vi "XboxControl.vi"() -> ()   [LabVIEW 2011]
uses:
  <vilib>/Utility/inputDevices.llb/joystickAcquire.vi
panel:
  out "A Speed Value":dbl
  in  "stop":bool
  out "direction info":T1
  out "button info":T2
  out "axis info":T3
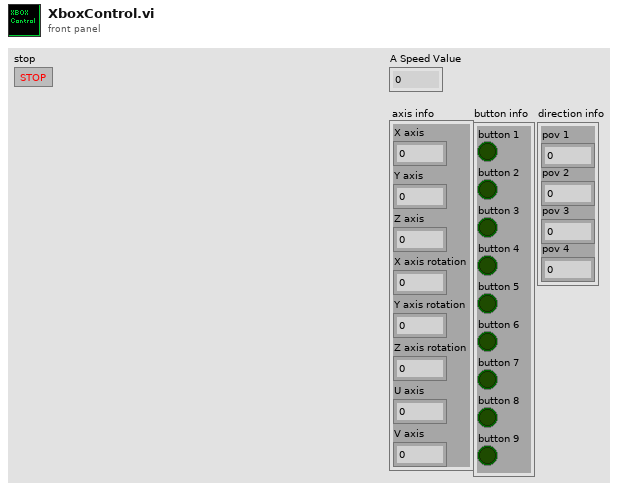
[diagram p1: front panel]
types:
  T1 = cluster{"pov 1":i32, "pov 2":i32, "pov 3":i32, "pov 4":i32}
  T2 = cluster{"button 1":bool, "button 2":bool, "button 3":bool, "button 4":bool, "button 5":bool, "button 6":bool, "button 7":bool, "button 8":bool, "button 9":bool, "button 10":bool, "button 11":bool, "button 12":bool, "button 13":bool, "button 14":bool, "button 15":bool, "button 16":bool, "button 17":bool, "button 18":bool, "button 19":bool, "button 20":bool, "button 21":bool, "button 22":bool, "button 23":bool, "button 24":bool, "button 25":bool, "button 26":bool, "button 27":bool, "button 28":bool, "button 29":bool, "button 30":bool, "button 31":bool, "button 32":bool}
  T3 = cluster{"X axis":i32, "Y axis":i32, "Z axis":i32, "X axis rotation":i32, "Y axis rotation":i32, "Z axis rotation":i32, "U axis":i32, "V axis":i32}
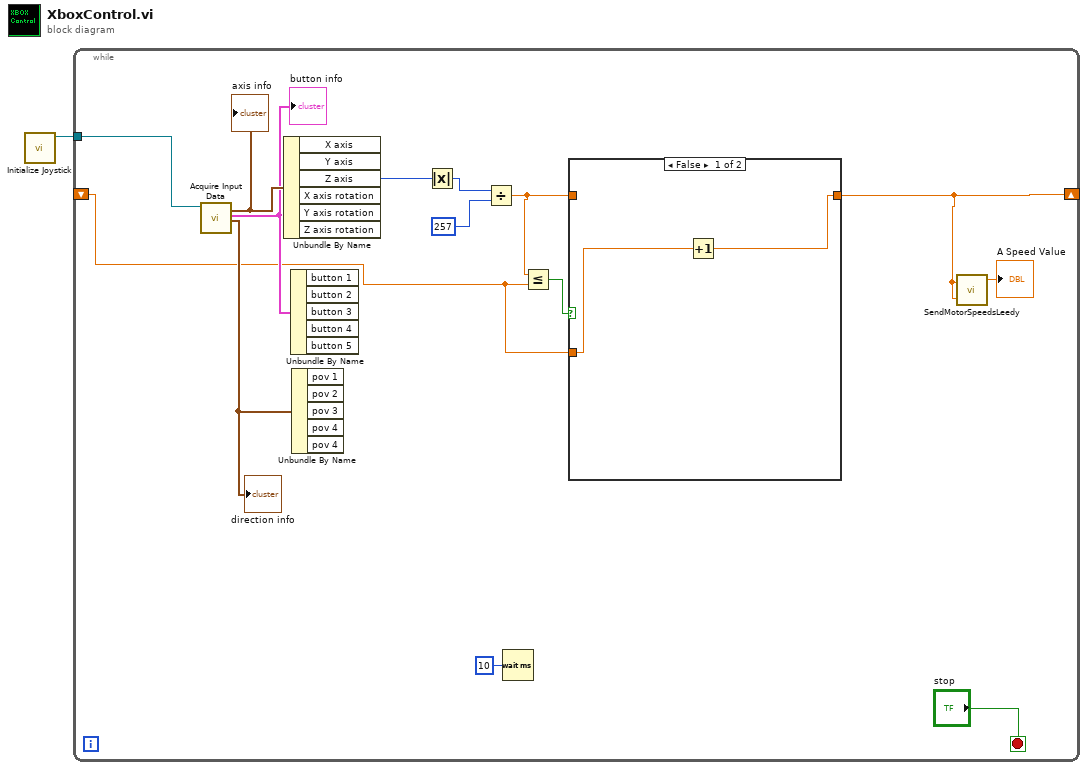
[diagram p0: block diagram]
diagram:
  n1 = call <vilib>:"Initialize Joystick.vi"() -> ("device ID"=w1:refnum<k1>)  [unwired: 10 in, 1 out]
  n2 = while {
    shift-right: [w3] -> _
    shift-left: _ -> [w5]
    tunnel: w1 -> [w4]
    stop <- "stop" stop-if-true
    n3 = call-poly <vilib>:"Acquire Input Data.vi"("device ID"=w4) -> ("axis info"=w15:T3, "button info"=w14:T2, "direction info"=w13:T1)  [unwired: 14 in, 2 out]
    "axis info" <- w15
    "button info" <- w14
    "direction info" <- w13
    n4 = Unbundle By Name(w15) -> ("Z axis"=w12:i32)  [unwired: 5 out]
    n5 = Unbundle By Name(w14) -> ()  [unwired: 5 out]
    n6 = Unbundle By Name(w13) -> ()  [unwired: 5 out]
    n7 = Absolute Value(x=w12) -> (abs(x)=w10:i32)
    n8 = Divide(x=w10, y=257) -> (x/y=w6:dbl)
    n9 = Wait (ms)(milliseconds to wait=u32 10) -> ()  [unwired: 1 out]
    n10 = Less Or Equal?(x=w6, y=w5) -> (x <= y?=w7:bool)
    n11 = case shown="False" w7 {
      tunnel: [w16 w18] -> w3
      tunnel: w6 -> [_ w18]
      tunnel: w5 -> [w17 _]
      frame False {
        n12 = Increment(x=w17) -> (x+1=w16:dbl)
      }
      frame True {
      }
    }
    n13 = call "SendMotorSpeedsLeedy.vi"("B Speed"=w3, "A Speed"=w3) -> ("A Speed Value"=→"A Speed Value":dbl)  [unwired: 4 out]
  }
